vi "sub_conv2ASV.vi"(11 "joystick info-out":T2) -> (3 "ASV_joystick":T1(array[cluster]))   [LabVIEW 2019]
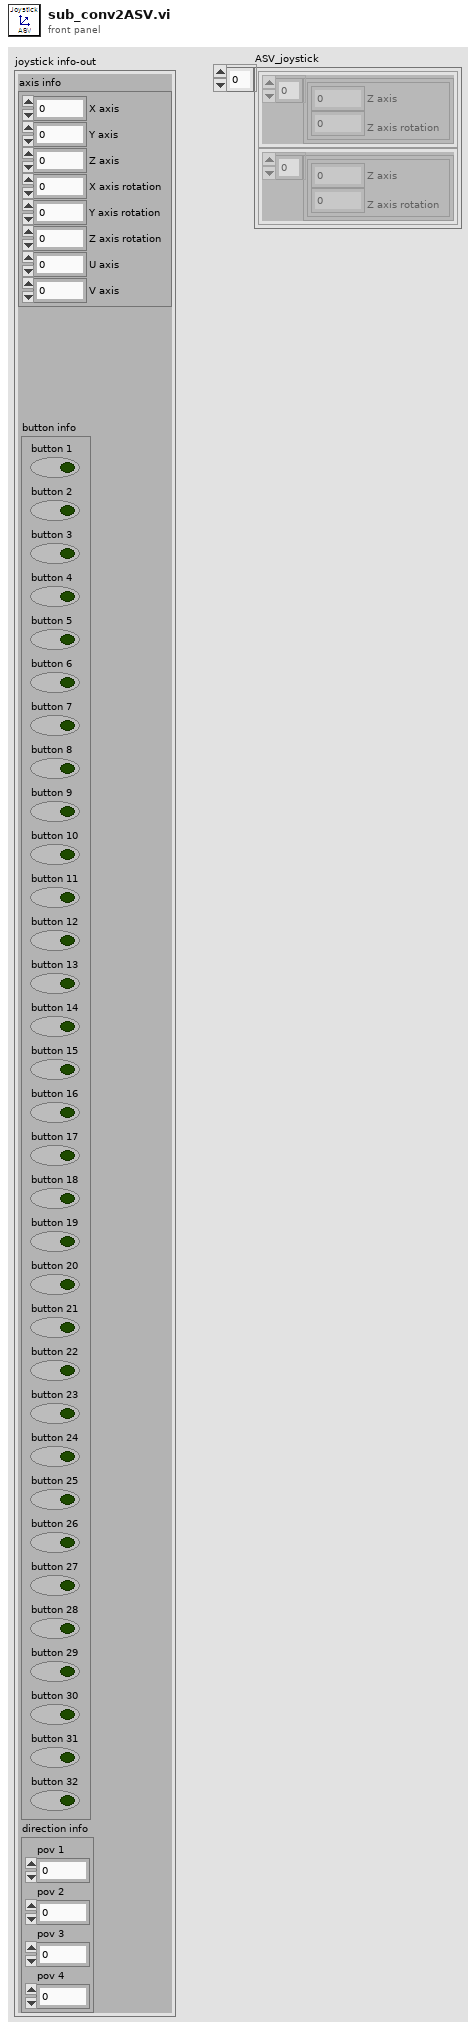
[diagram p1: front panel]
types:
  T1 = cluster{cluster{"Z axis":dbl, "Z axis rotation":dbl}[]}[]
  T2 = cluster{"axis info":cluster{"X axis":i32, "Y axis":i32, "Z axis":i32, "X axis rotation":i32, "Y axis rotation":i32, "Z axis rotation":i32, "U axis":i32, "V axis":i32}, "button info":cluster{"button 1":bool, "button 2":bool, "button 3":bool, "button 4":bool, "button 5":bool, "button 6":bool, "button 7":bool, "button 8":bool, "button 9":bool, "button 10":bool, "button 11":bool, "button 12":bool, "button 13":bool, "button 14":bool, "button 15":bool, "button 16":bool, "button 17":bool, "button 18":bool, "button 19":bool, "button 20":bool, "button 21":bool, "button 22":bool, "button 23":bool, "button 24":bool, "button 25":bool, "button 26":bool, "button 27":bool, "button 28":bool, "button 29":bool, "button 30":bool, "button 31":bool, "button 32":bool}, "direction info":cluster{"pov 1":i32, "pov 2":i32, "pov 3":i32, "pov 4":i32}}
  T3 = cluster{"X axis":i32, "Y axis":i32, "Z axis":i32, "X axis rotation":i32, "Y axis rotation":i32, "Z axis rotation":i32, "U axis":i32, "V axis":i32}
  T4 = cluster{cluster{"Z axis":dbl, "Z axis rotation":dbl}[]}
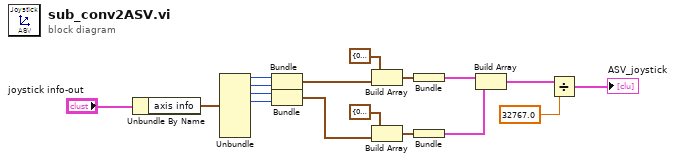
[diagram p0: block diagram]
diagram:
  n1 = Unbundle By Name("joystick info-out") -> ("axis info"=w8:T3)
  n2 = Unbundle(w8) -> ("X axis"=w7:i32, "Y axis"=w6:i32, "Z axis"=w5:i32, "Z axis rotation"=w4:i32)  [unwired: 4 out]
  n3 = Bundle("X axis"=w7, "Y axis"=w6) -> (w13:cluster{"X axis":i32, "Y axis":i32})  [unwired: 1 in]
  n4 = Bundle("Z axis"=w5, "Z axis rotation"=w4) -> (w10:cluster{"Z axis":i32, "Z axis rotation":i32})  [unwired: 1 in]
  n5 = Build Array(cluster{dbl, dbl} {0.0, 0.0} ("element"), w13) -> (w15:cluster{"X axis":dbl, "Y axis":dbl}[])
  n6 = Build Array(cluster{dbl, dbl} {0.0, 0.0} ("element"), w10) -> (w12:cluster{"Z axis":dbl, "Z axis rotation":dbl}[])
  n7 = Bundle(w15) -> (w14:cluster{cluster{"X axis":dbl, "Y axis":dbl}[]})  [unwired: 1 in]
  n8 = Bundle(w12) -> (w9:T4)  [unwired: 1 in]
  n9 = Build Array(w14, w9) -> (w2:T1)
  n10 = Divide(x=w2, y=32767.0) -> (x/y=→"ASV_joystick":T1)
